vi "加载要求值到报表.vi"(6 "油动机名称":string, 8 "error out 4":errorcluster caption="error out", 9 "试验表格refnum in":T1, 10 "错误输入（无错误）":errorcluster caption="error out", 11 "要求值表格refnum in":T1) -> (0 "error out":errorcluster, 1 "试验表格refnum out":T1, 2 "错误输出":errorcluster caption="error out", 3 "要求值表格refnum out":T1)   [LabVIEW 2013]
uses:
  <vilib>/Utility/config.llb/Config Data RefNum.ctl
  <vilib>/Utility/config.llb/Read Key (String).vi
  <vilib>/Utility/config.llb/Write Key (String).vi
  <vilib>/Utility/config.llb/NI_LVConfig.lvlib
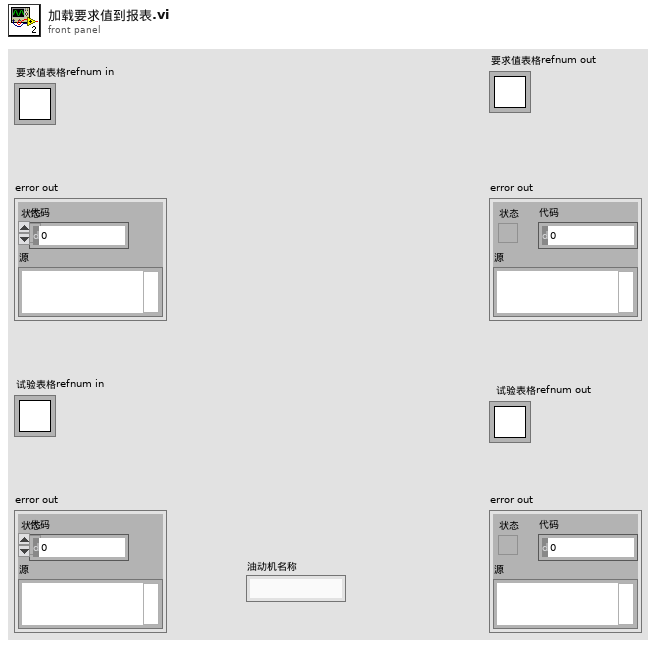
[diagram p1: front panel]
types:
  T1 = typedef "NI_LVConfig.lvlib/Config Data RefNum.ctl" = refnum<k1>
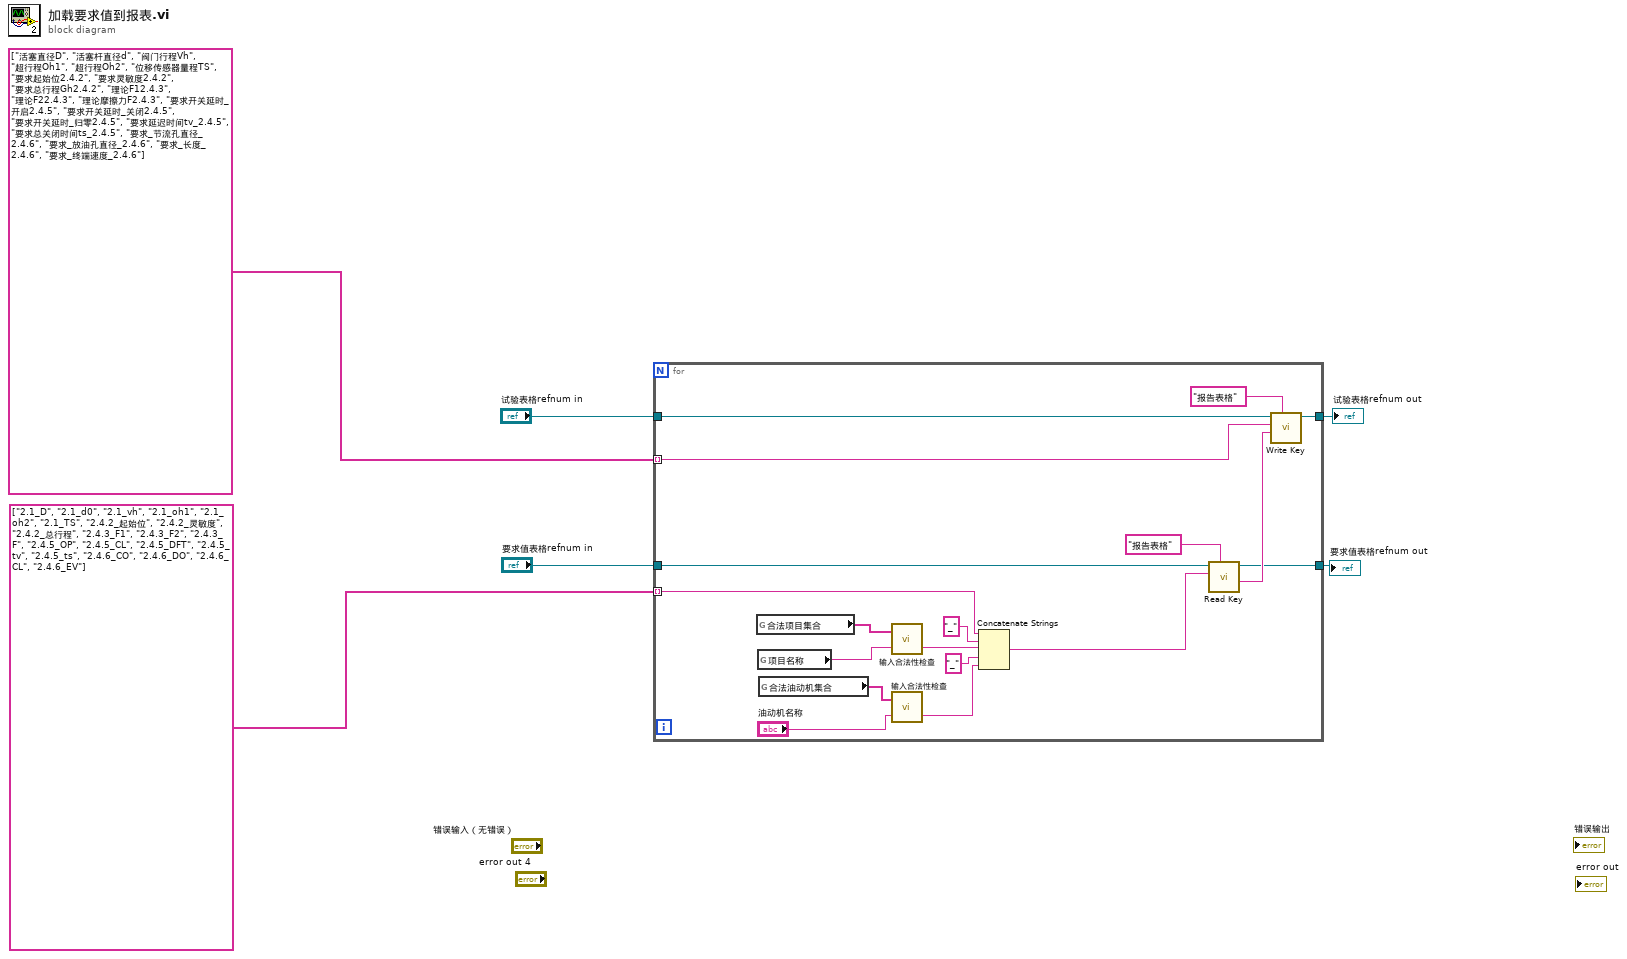
[diagram p0: block diagram]
diagram:
  n1 = for {
    tunnel: "要求值表格refnum in" -> [w23]
    tunnel: "试验表格refnum in" -> [w20]
    tunnel: string[] ["活塞直径D", "活塞杆直径d", "阀门行程Vh", "超行程Oh1", "超行程Oh2", "位移传感器量程TS", "要求起始位2.4.2", "要求灵敏度2.4.2", "要求总行程Gh2.4.2", "理论F12.4.3", "理论F22.4.3", "理论摩擦力F2.4.3", "要求开关延时_开启2.4.5", "要求开关延时_关闭2.4.5", "要求开关延时_归零2.4.5", "要求延迟时间tv_2.4.5", "要求总关闭时间ts_2.4.5", "要求_节流孔直径_2.4.6", "要求_放油孔直径_2.4.6", "要求_长度_2.4.6", "要求_终端速度_2.4.6"] -> [w11] mode=indexing
    tunnel: [w18] -> w5
    tunnel: [w17] -> w6
    tunnel: string[] ["2.1_D", "2.1_d0", "2.1_vh", "2.1_oh1", "2.1_oh2", "2.1_TS", "2.4.2_起始位", "2.4.2_灵敏度", "2.4.2_总行程", "2.4.3_F1", "2.4.3_F2", "2.4.3_F", "2.4.5_OP", "2.4.5_CL", "2.4.5_DFT", "2.4.5_tv", "2.4.5_ts", "2.4.6_CO", "2.4.6_DO", "2.4.6_CL", "2.4.6_EV"] -> [w10] mode=indexing
    n2 = global read "合法项目集合.vi" "合法项目集合"() -> (w16:string[])
    n3 = global read "项目名称.vi" "项目名称"() -> (w15:string)
    n4 = global read "合法油动机集合.vi" "合法油动机集合"() -> (w13:string[])
    n5 = call "输入合法性检查.vi"("被检查名称"=w15, "合法名称集合"=w16) -> ("合法名称"=w14:string)  [unwired: 1 out]
    n6 = call "输入合法性检查.vi"("被检查名称"="油动机名称", "合法名称集合"=w13) -> ("合法名称"=w8:string)  [unwired: 1 out]
    n7 = Concatenate Strings(w10, "_" ("字符串"), w14, "_" ("字符串"), w8) -> (w7:string)
    n8 = call-poly <vilib>:"Read Key.vi"("section"="报告表格", "key"=w7, "refnum"=w23) -> ("value"=w19:string, "refnum out"=w17:T1)  [unwired: 5 in, 2 out]
    n9 = call-poly <vilib>:"Write Key.vi"("section"="报告表格", "value"=w19, "key"=w11, "refnum"=w20) -> ("refnum out"=w18:T1)  [unwired: 5 in, 2 out]
  }
  "要求值表格refnum out" <- w6
  "试验表格refnum out" <- w5
